vi "RT Global References.vi"() -> ()   [LabVIEW 2015]
panel:
  in  "RT Loop STOP":bool
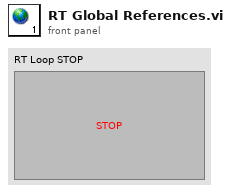
[diagram p1: front panel]
diagram:
